vi "One_Ball_Auto.vi"(0 "Cam_Angle_To_Target":dbl=2.0715725691444784, 1 "Stopped":bool=TRUE, 2 "Dist to target":dbl=13.335309538727138, 3 "Auto_Control":T1=enum."One  Ball", 4 "Encoder_Left":dbl=-219.798918, 6 "Ultra_Sonic_Dist":dbl=31.344557836190454, 10 "Auto_Enable":bool, 14 "Yaw":dbl=63.921912939715384, 15 "Aimed?":bool) -> (18 "Intake Arm Lowered":bool, 19 "Drive_FWD Speed":dbl, 20 "Angle_Setpoint":dbl, 21 "Stage":bool, 22 "Drive_Enable":bool, 23 "Shoot":bool, 24 "Auto_Aim":bool, 25 "Rest_Encoder":bool, 26 "Rest_Gyro":bool, 27 "One_Ball_Auto":bool)   [LabVIEW 2015]
uses:
  One_Ball_Type_Def.ctl
  Auto_Selection.ctl
panel:
  in  "Ramp_Rate":dbl=1.2 format="%#_13g"
  in  "DriveForward_TIme out":i32=10000
  in  "Turning_Timeout":i32=2000
  in  "DRive to shoot time out":i32=5000
  in  "Drive_to_shoot":dbl=-0.2 format="%#_13g"
  in  "DRive_Forward_1":dbl=-1.0 format="%#_13g"
  in  "Yaw Delta Error":dbl=5.0
  in  "Max_Dist_to_Def":dbl=65.0
  in  "Min_Dist_to_Def":dbl=25.0
  out "State":T2=enum."off"
  out "error":errorcluster={"status"=TRUE, "code"=0, "source"="Drive to Shoot: Test Stop"}
  in  "Stop_DB":dbl=4.0 format="%#_13g"
  in  "Test_Stop_State":T2=enum."Drive to Shoot"
  in  "Dist_Stop_Before_Target":dbl=50.0 format="%#_13g"
  in  "Angle Turn_to_targe_DB":dbl=20.0 format="%#_13g"
  in  "Angle Turn_to_target_delta":dbl=0.5
  in  "Angle Turn_to_target":dbl=-60.0 format="%#_13g"
  in  "Dist_Low_Bar_to_Turn":dbl=160.0 format="%#_13g"
  in  "Dist_to_Lower_Arm":dbl=36.0 format="%#_13g"
  in  "Clear Error":bool
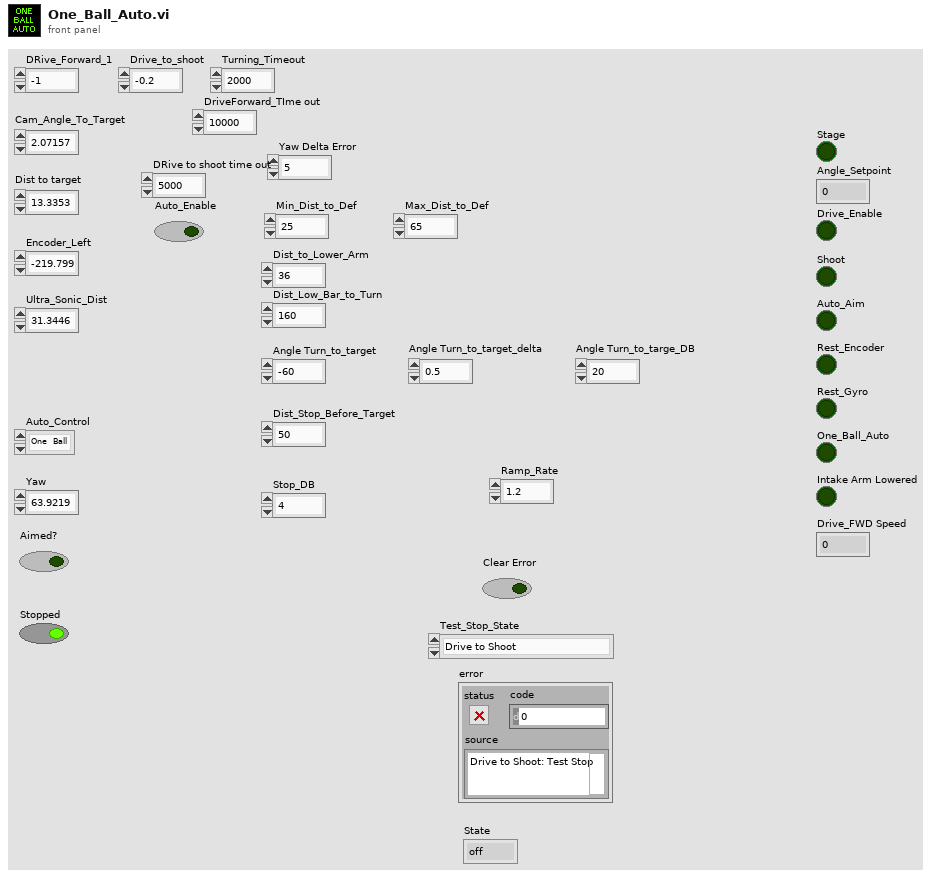
[diagram p1: front panel]
types:
  T1 = typedef "Auto_Selection.ctl" = enum16{"Low Bar", "Rough Terrain", "Rock Wall", "Ramparts", "Moat", "Cheval de Frise", "Portcullis", "None", "One  Ball", "Shoot"}
  T2 = typedef "One_Ball_Type_Def.ctl" = enum16{"Stop", "DriveForward", "LowerArm", "BeforeTeeter", "ResetOff", "ResetVar", "off", "Stop One", "Stop Two", "Tunr 60 deg", "Find Target", "Drive to Shoot", "Turn to target", "Shoot", "Stop Three", "Stop_After_Aim"}
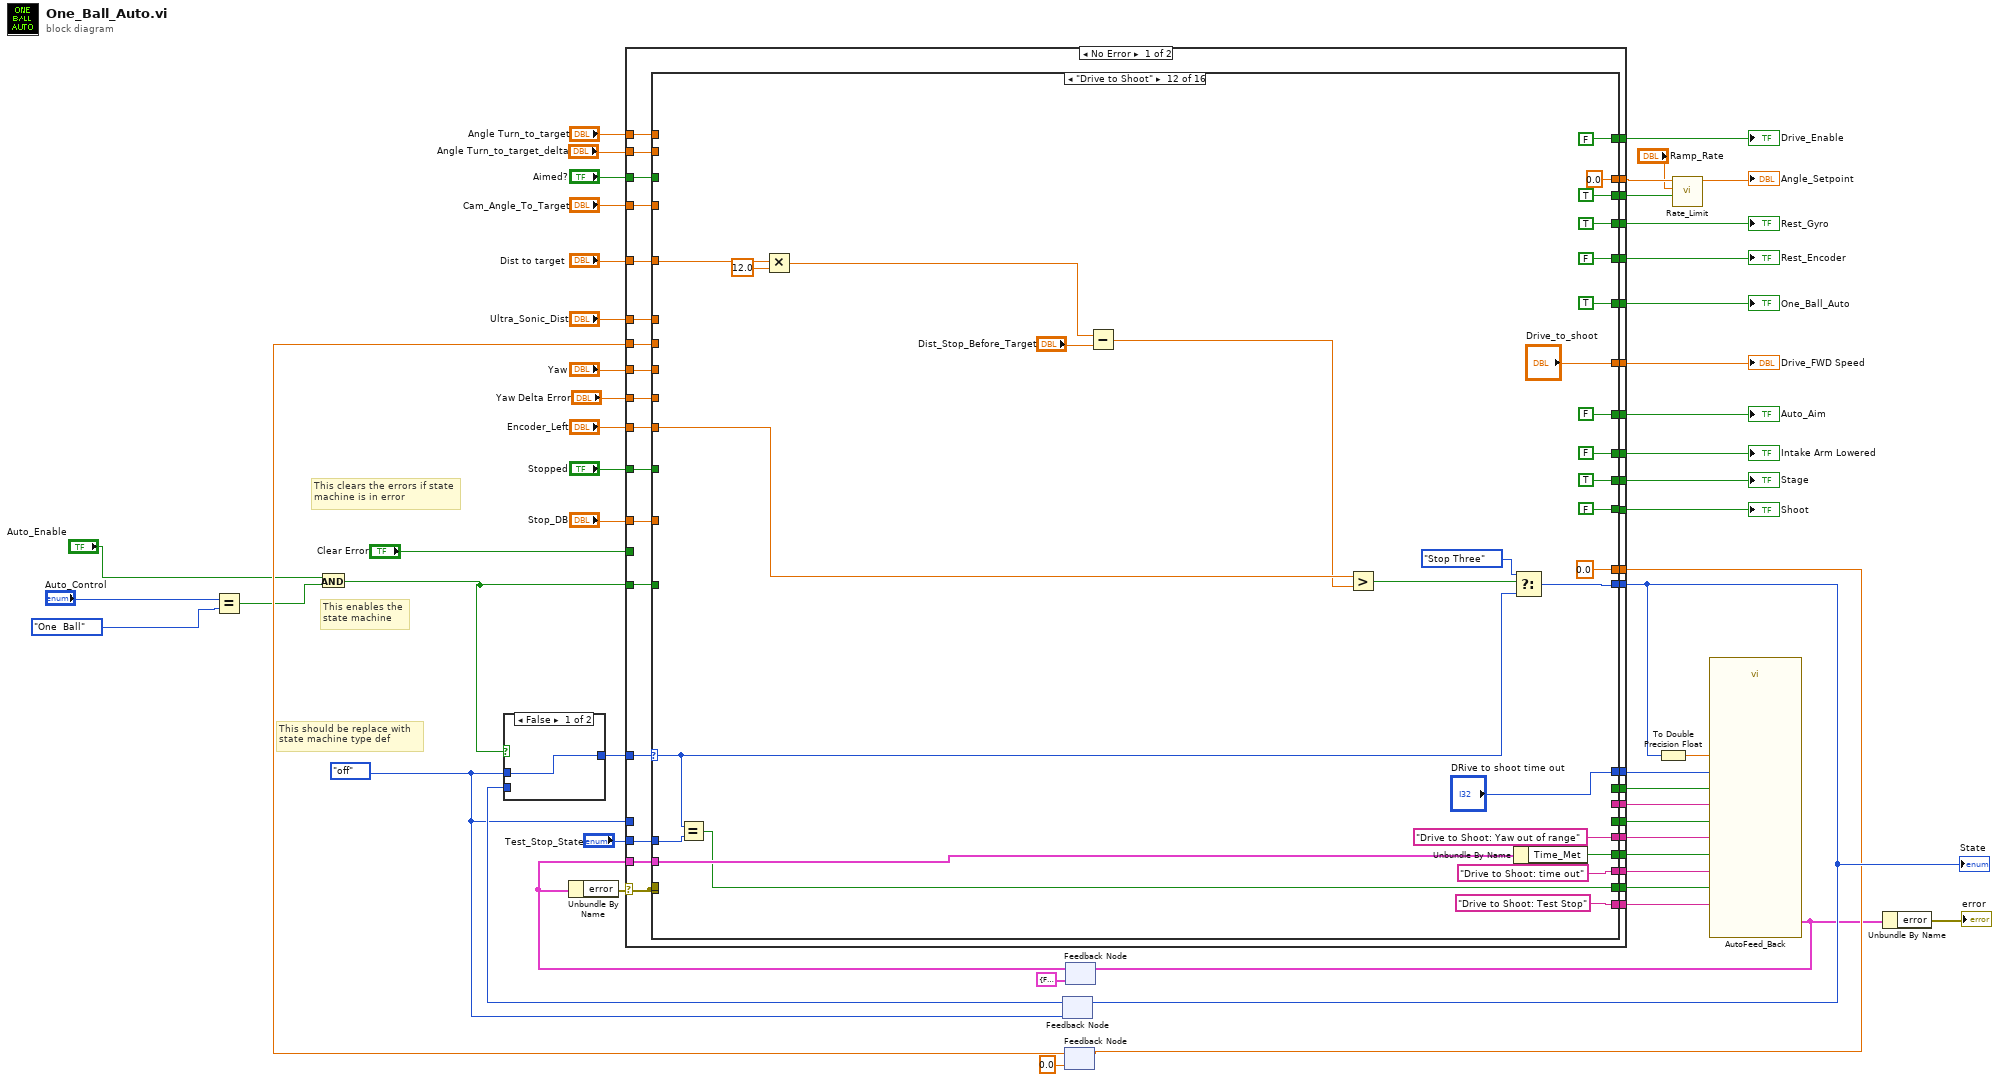
[diagram p0: block diagram]
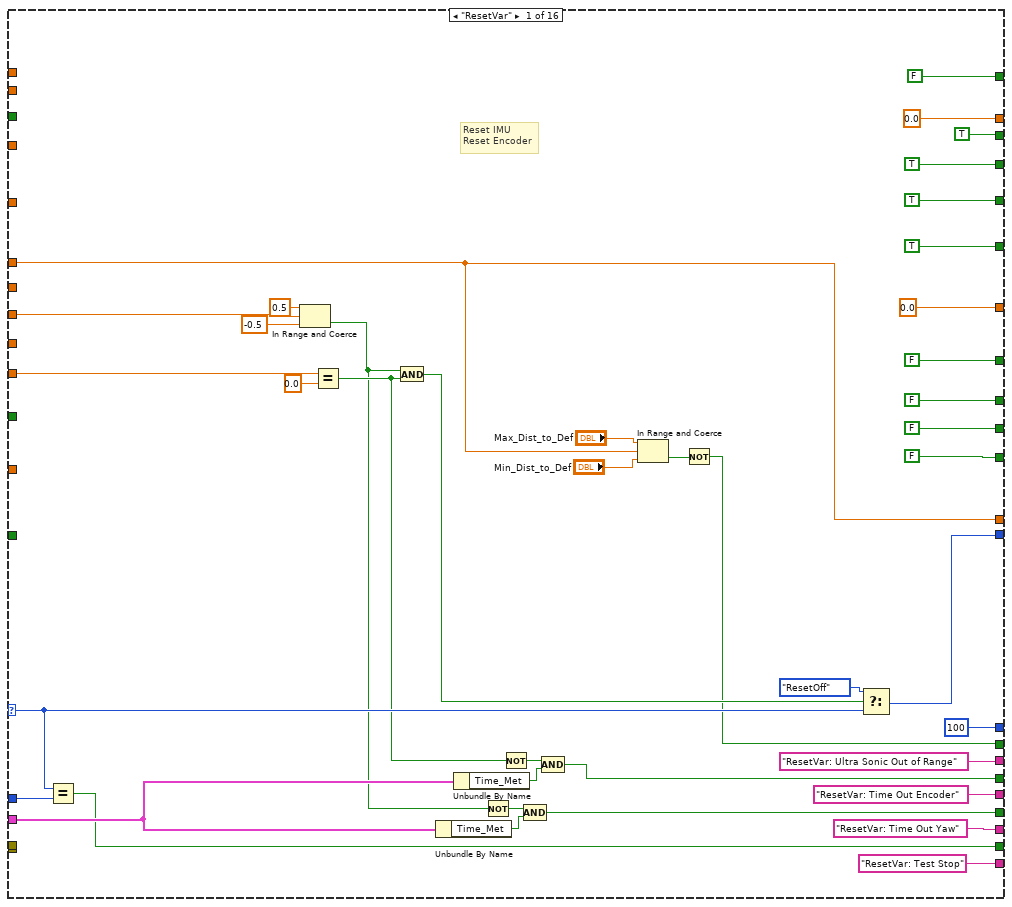
[diagram p3: hidden frame]
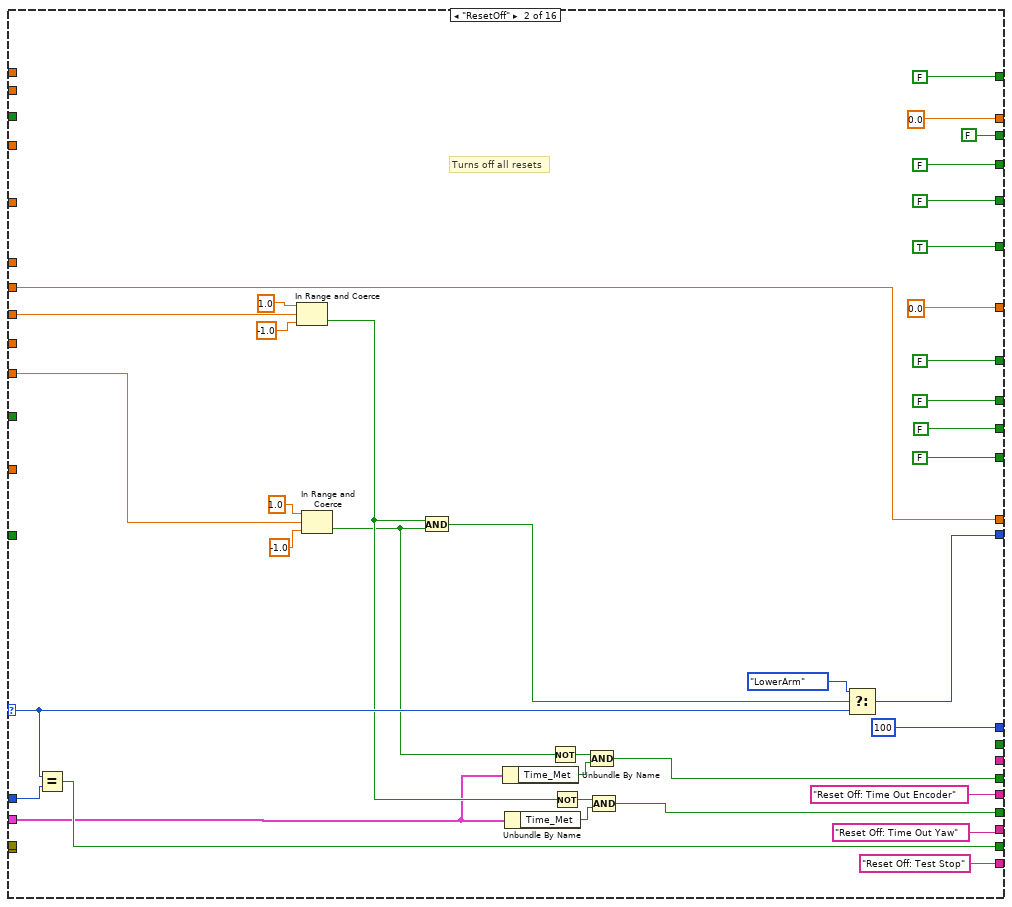
[diagram p4: hidden frame]
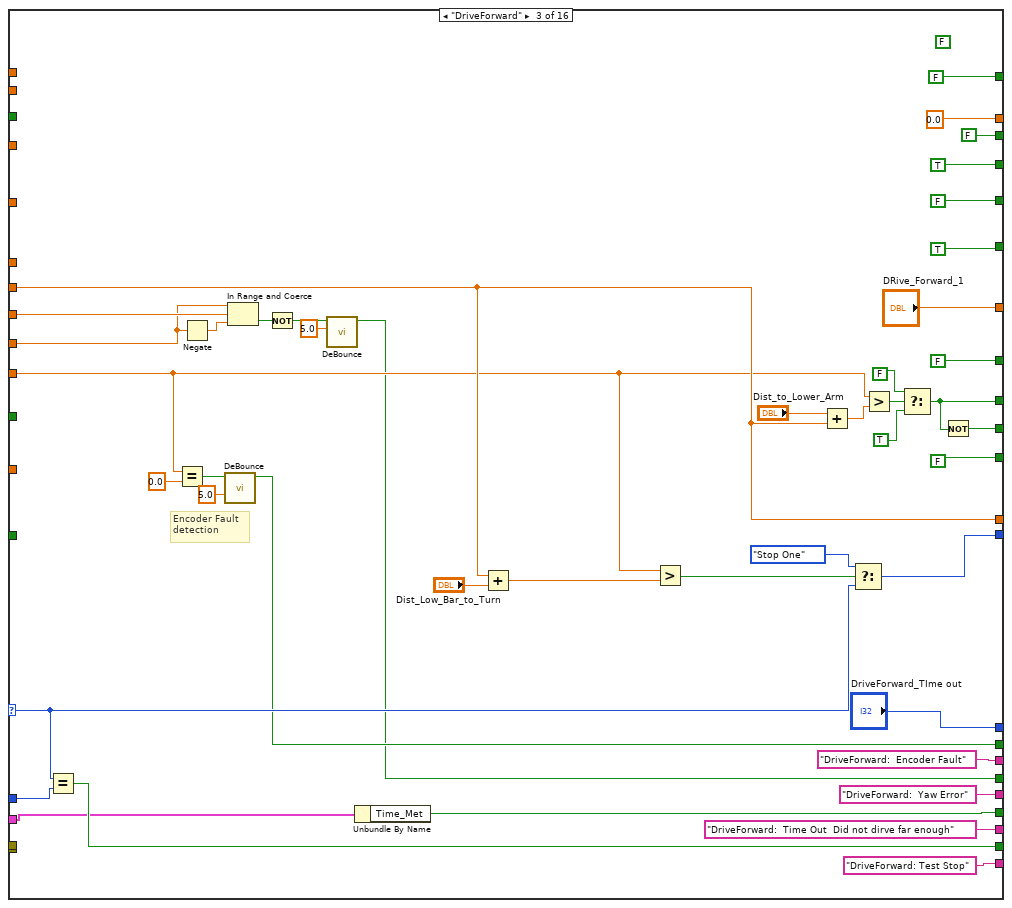
[diagram p5: hidden frame]
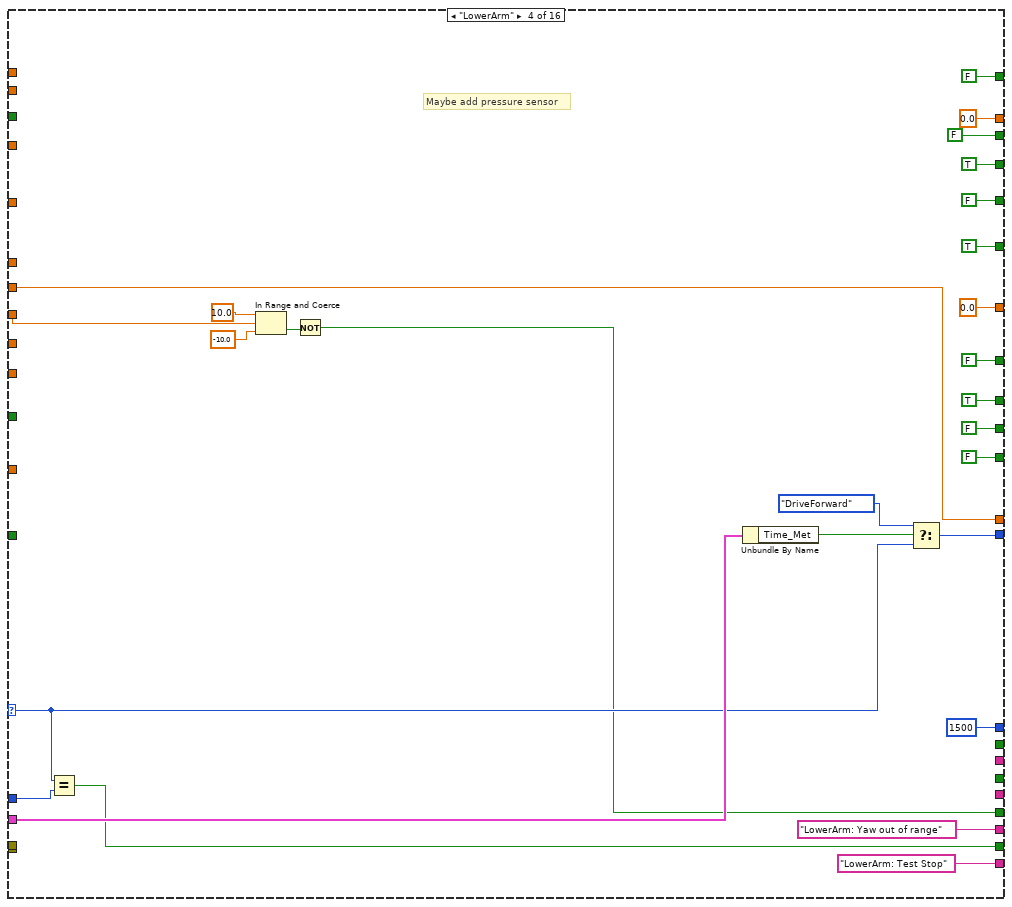
[diagram p6: hidden frame]
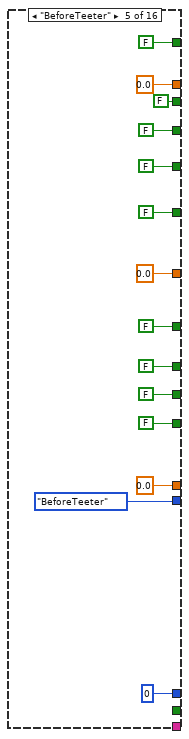
[diagram p7: hidden frame]
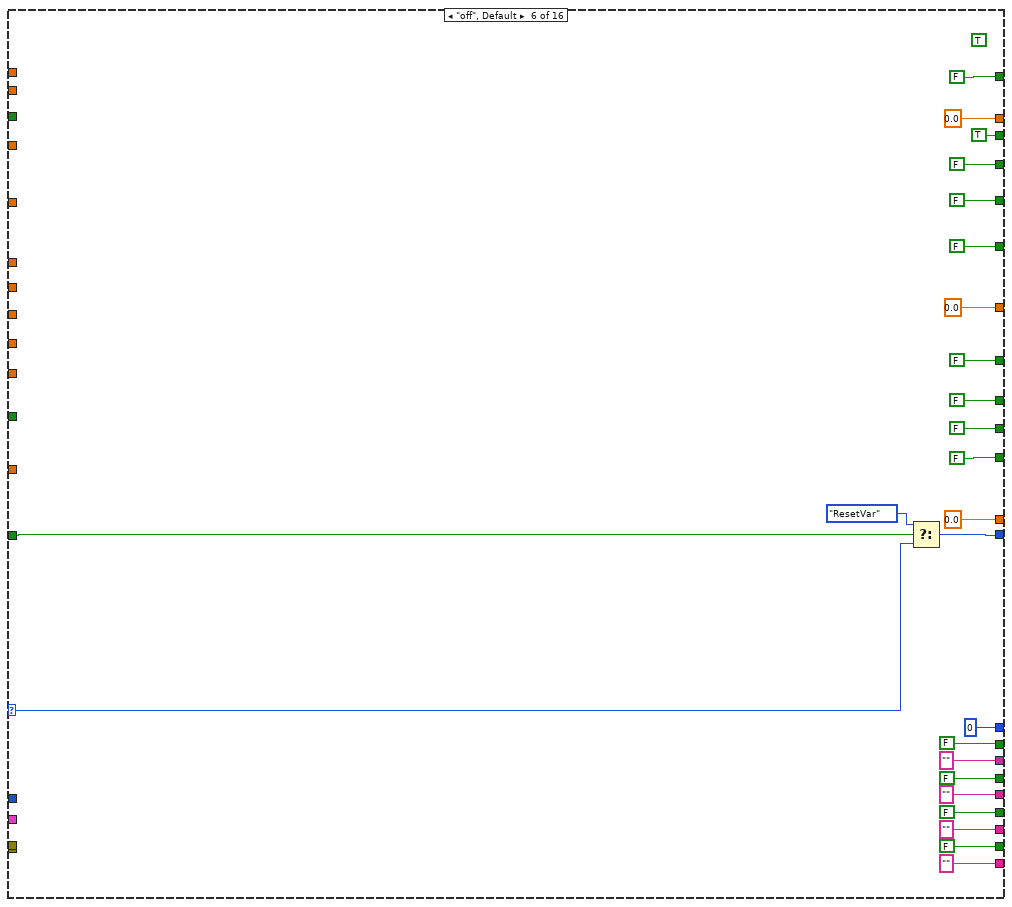
[diagram p8: hidden frame]
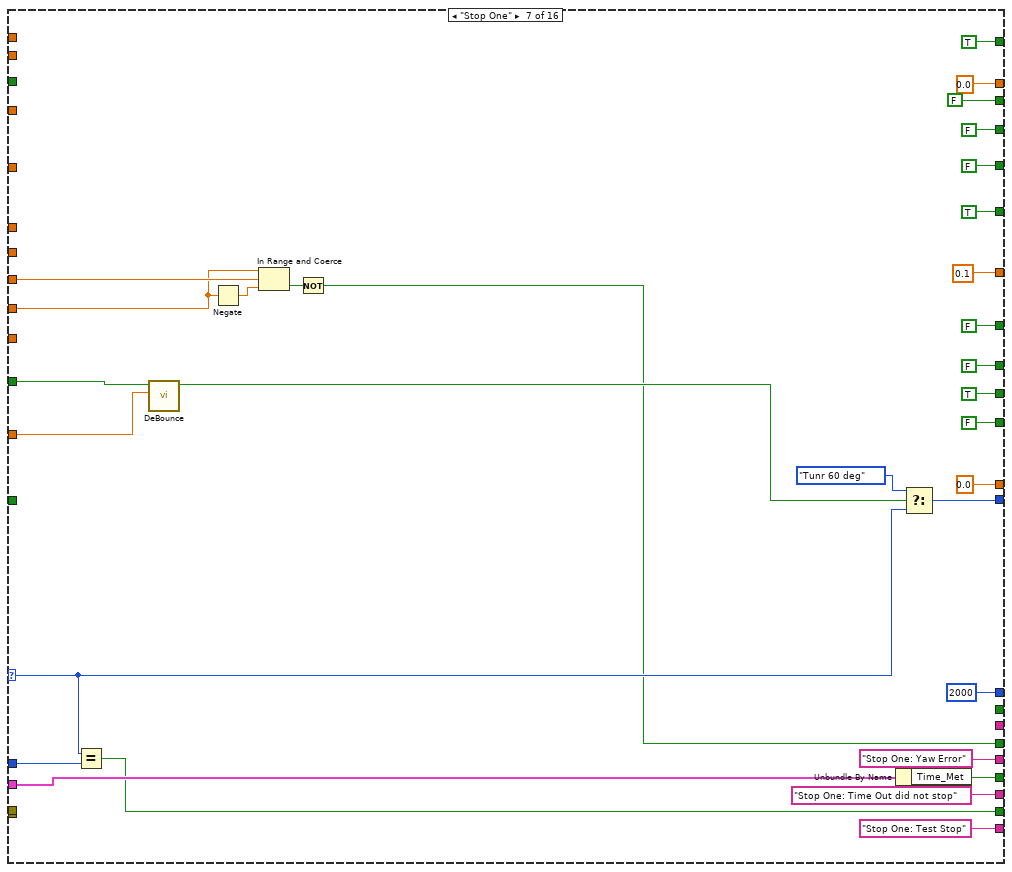
[diagram p9: hidden frame]
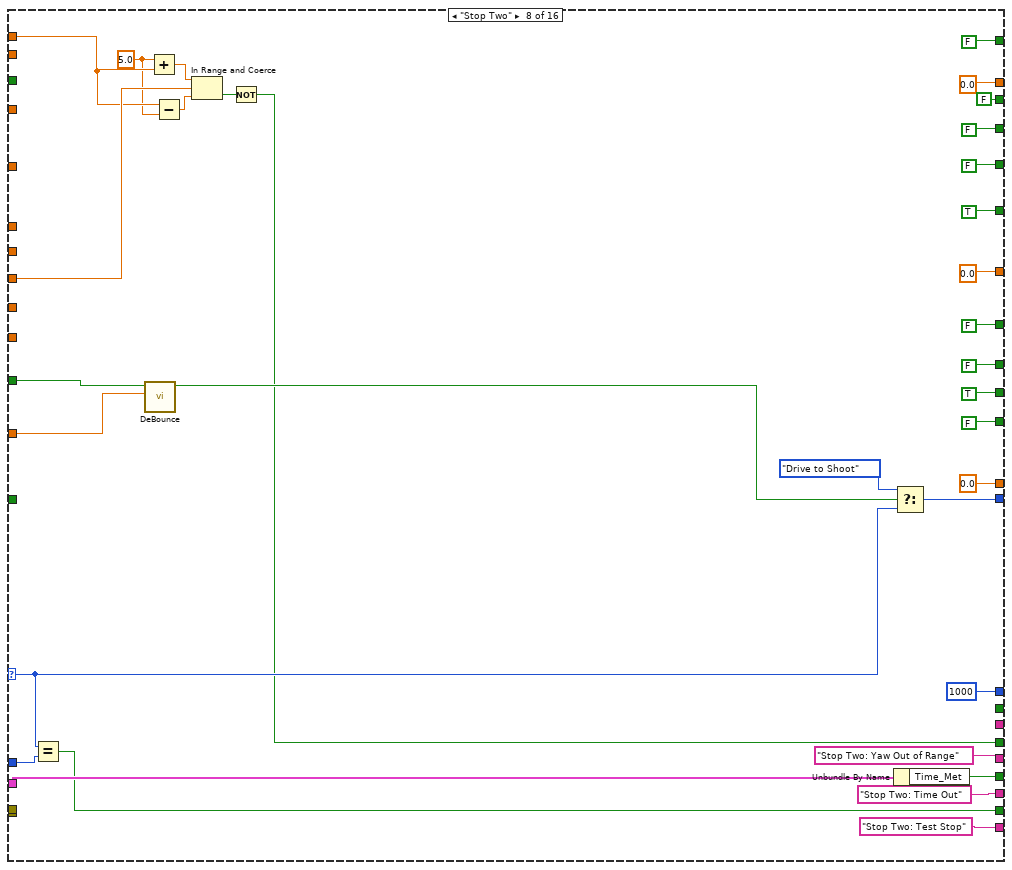
[diagram p10: hidden frame]
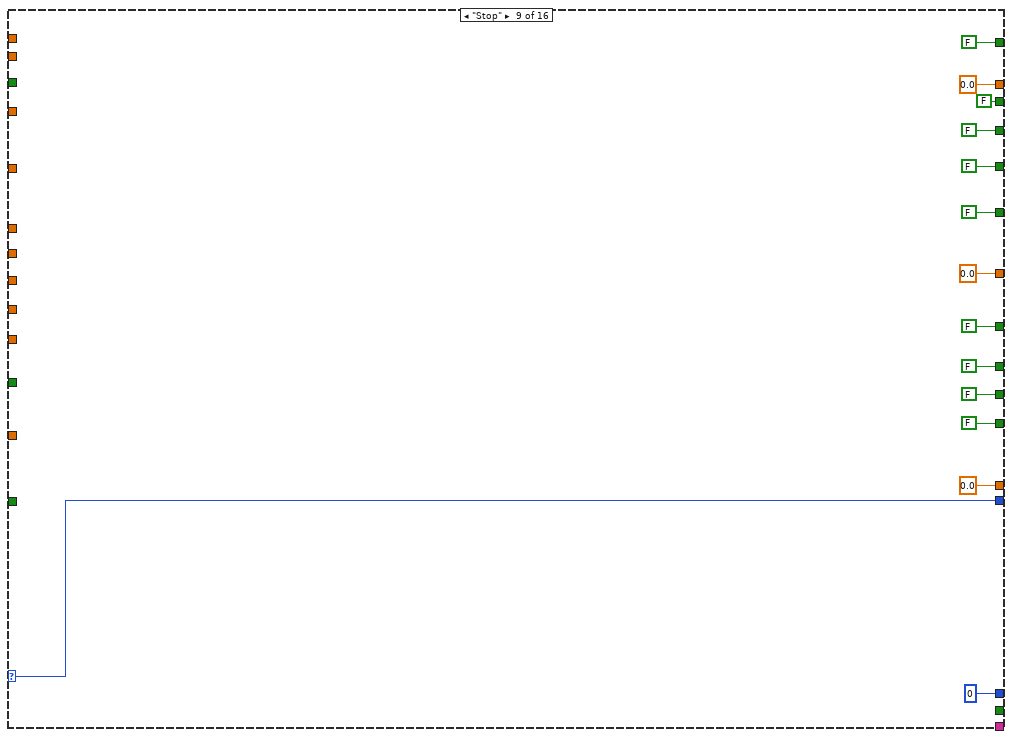
[diagram p11: hidden frame]
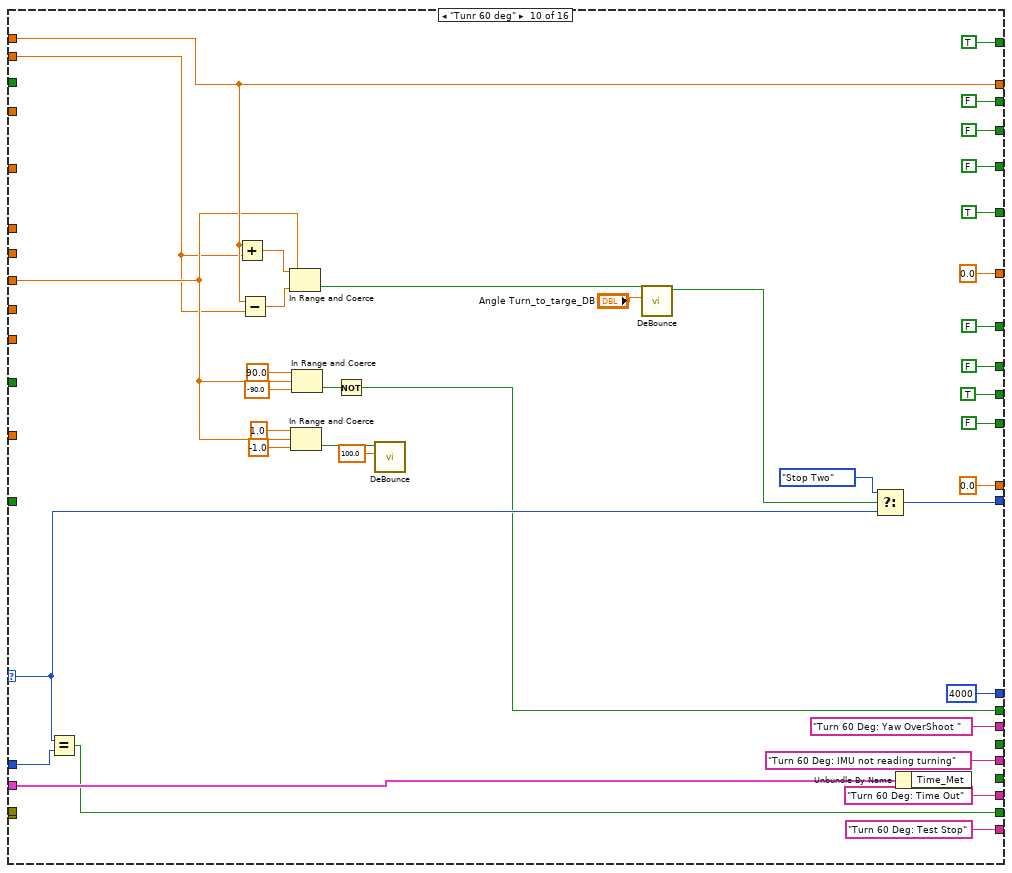
[diagram p12: hidden frame]
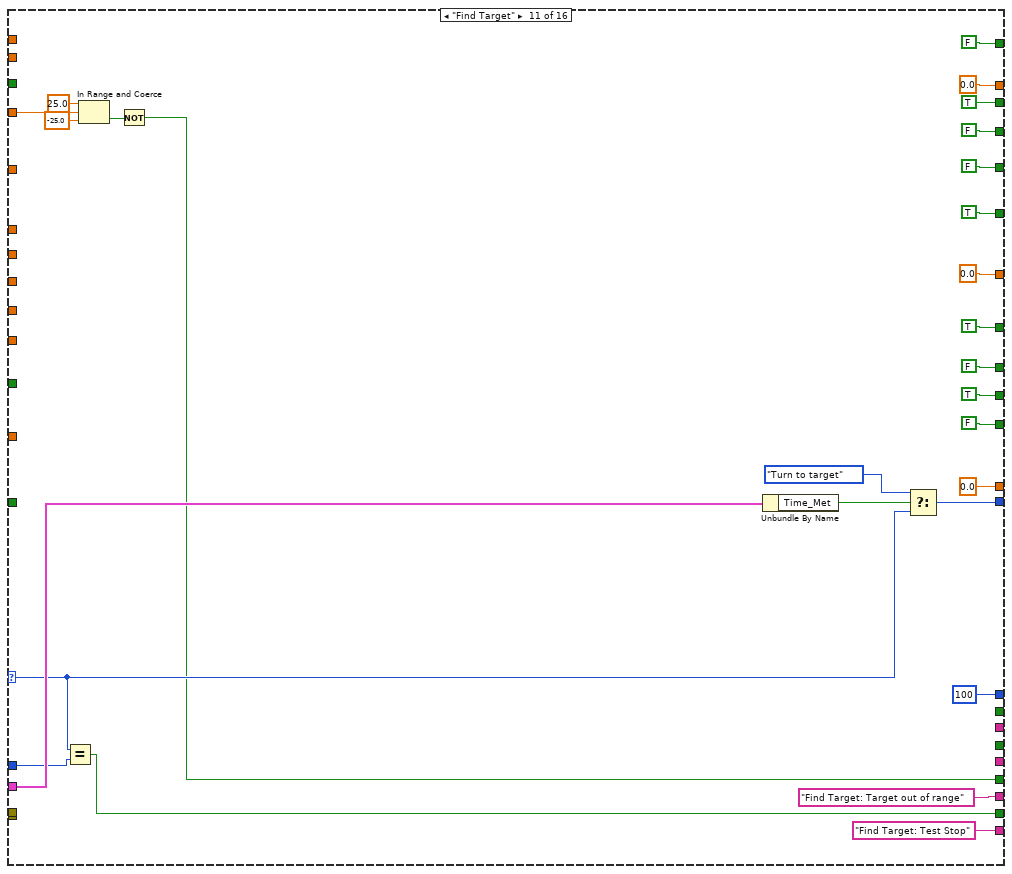
[diagram p13: hidden frame]
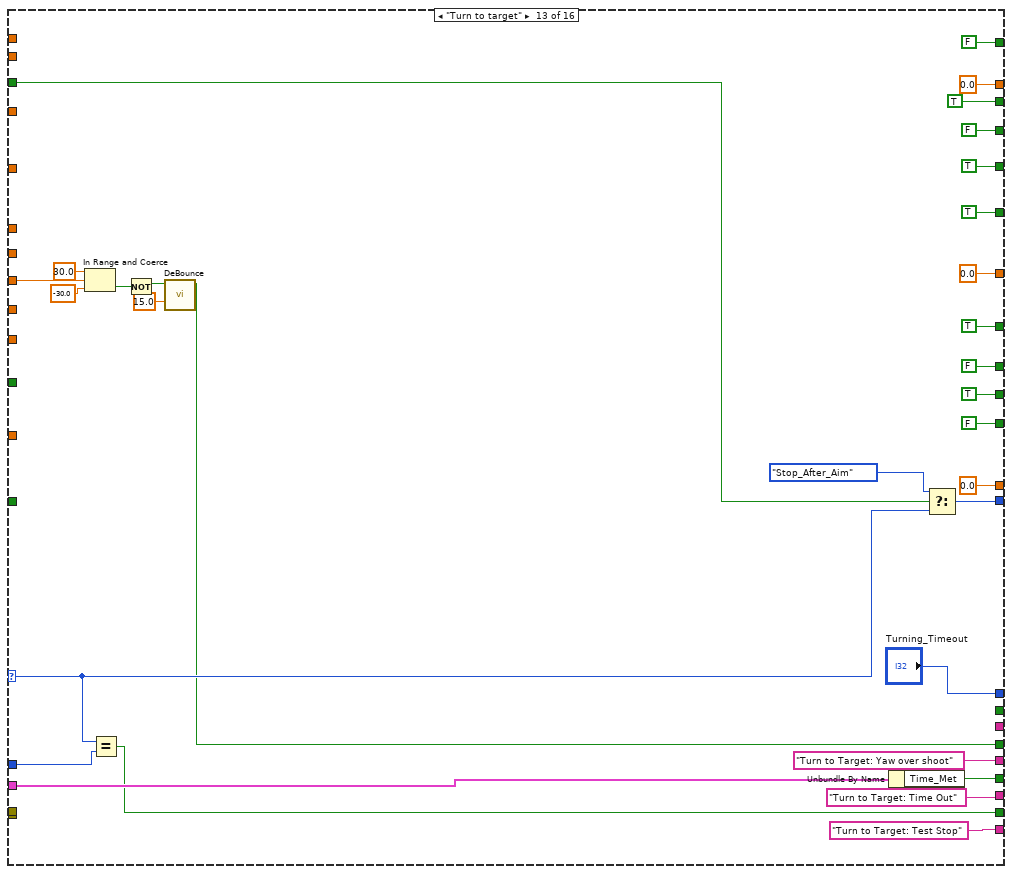
[diagram p14: hidden frame]
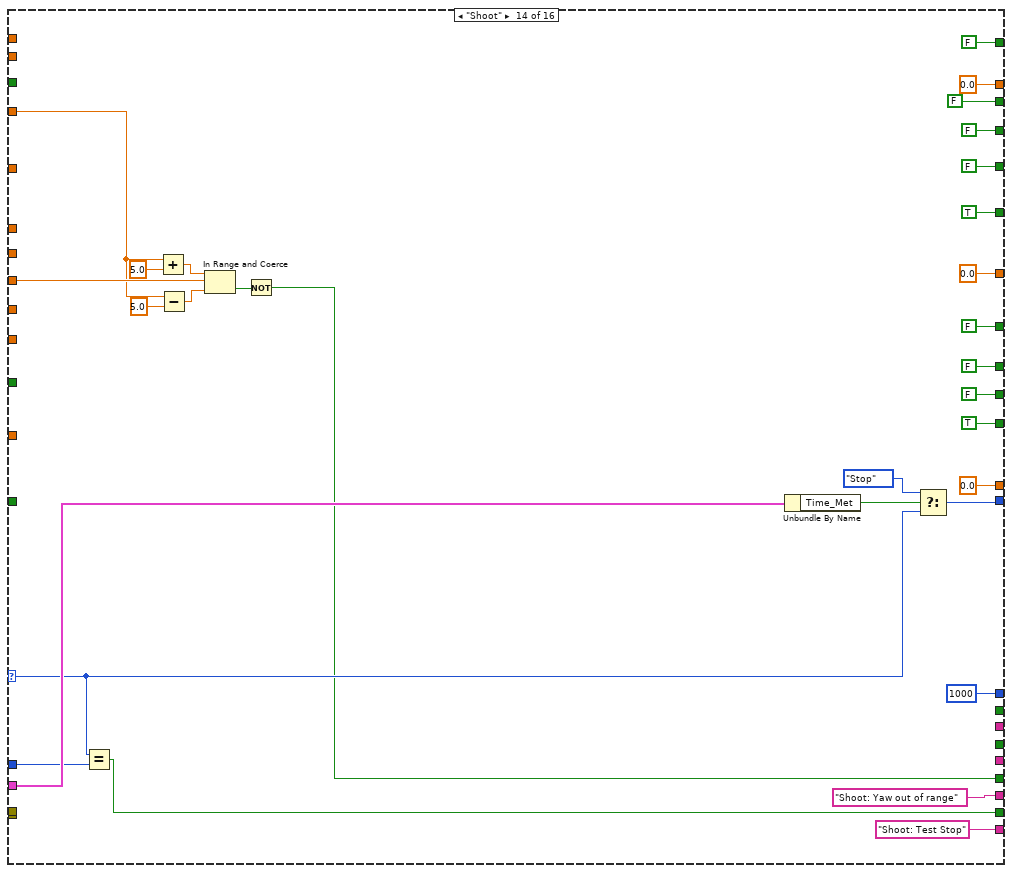
[diagram p15: hidden frame]
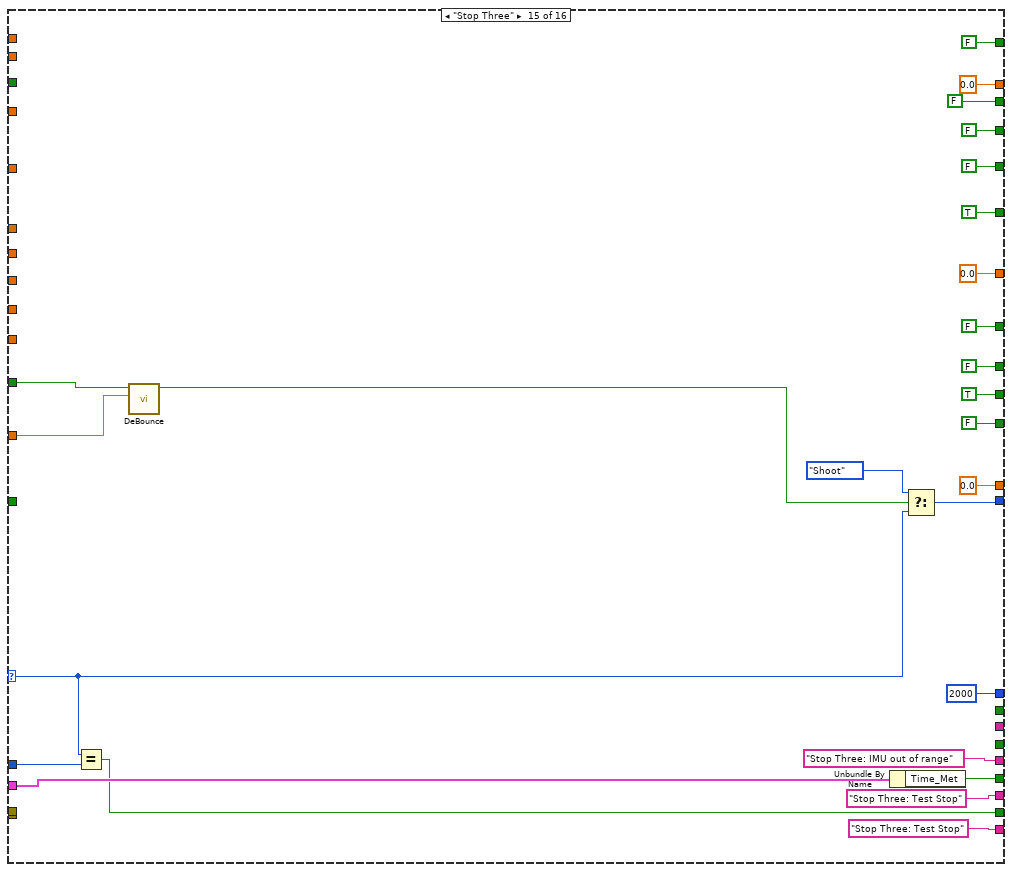
[diagram p16: hidden frame]
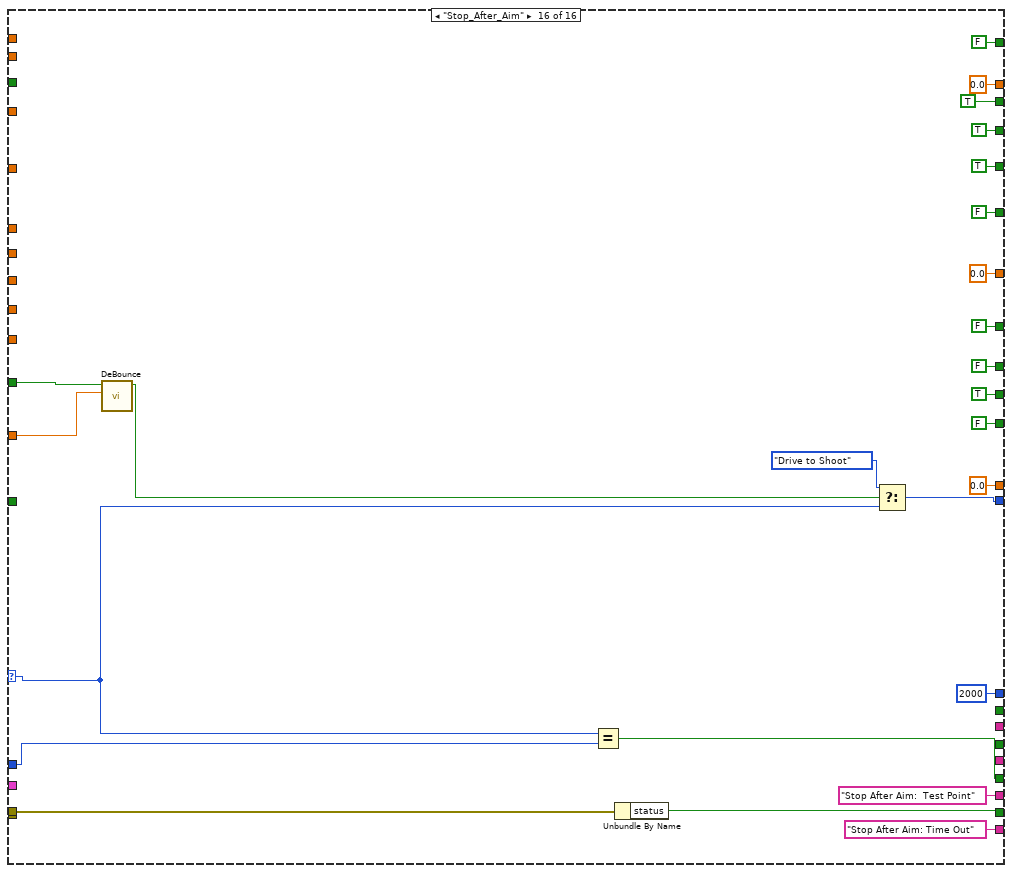
[diagram p17: hidden frame]
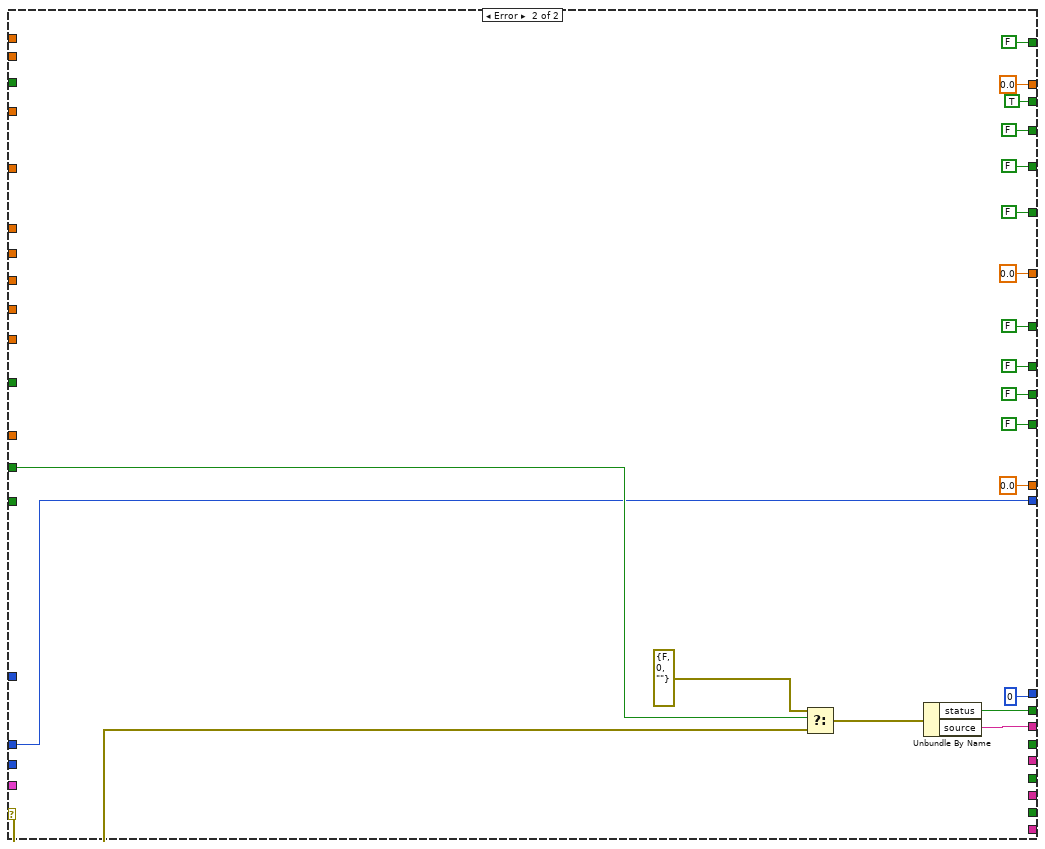
[diagram p18: hidden frame]
diagram:
  w33 = One_Ball_Type_Def."off"
  # "This clears the errors if state \nmachine is in error"
  # "This enables the \nstate machine"
  # "This should be replace with \nstate machine type def"
  n1 = Equal?(x="Auto_Control", y=Auto_Selection."One  Ball" ("Auto_Contorl.Auto_Selection 2")) -> (x = y?=w5:bool)
  n2 = And(x="Auto_Enable", y=w5) -> (x .and. y?=w3:bool)
  n3 = feedback #1(w33) -> (w45:T2)
  n4 = case shown="False" w3 {
    tunnel: w33 -> [w54 _]
    tunnel: [w54 w55] -> w46
    tunnel: w45 -> [_ w55]
    frame False {
    }
    frame True {
    }
  }
  n5 = feedback #2(0.0 ("Forward_Dist")) -> (w26:dbl)
  n6 = feedback #3(cluster{"Time_Met":bool, "error ":errorcluster} {"Time_Met"=FALSE, "error "={"status"=FALSE, "code"=0, "source"=""}} ("Feedback_State")) -> (w47:cluster{"Time_Met":bool, "error ":errorcluster})
  n7 = Unbundle By Name(w47) -> ("error"=w49:errorcluster)
  n8 = case shown="No Error" w49 {
    selector: w49 -> [w56 w572]
    tunnel: [w94 FALSE] -> w53
    tunnel: [w93 FALSE] -> w52
    tunnel: [w92 w585] -> w38
    tunnel: [w91 0] -> w51
    tunnel: "Clear Error" -> [_ w586]
    tunnel: w47 -> [w90 _]
    tunnel: w3 -> [w89 _]
    tunnel: w46 -> [w78 _]
    tunnel: w33 -> [_ w585]
    tunnel: [w88 0.0] -> w43
    tunnel: [w87 FALSE] -> w42
    tunnel: [w86 FALSE] -> w41
    tunnel: "Yaw" -> [w85 _]
    tunnel: "Encoder_Left" -> [w84 _]
    tunnel: [w83 FALSE] -> w37
    tunnel: [w82 FALSE] -> w36
    tunnel: "Ultra_Sonic_Dist" -> [w81 _]
    tunnel: [w80 0.0 ("Forward_Dist")] -> w22
    tunnel: w26 -> [w79 _]
    tunnel: [w77 0.0 ("Angle Turn_to_target")] -> w2
    tunnel: [w76 FALSE] -> w32
    tunnel: [w75 FALSE] -> w31
    tunnel: "Dist to target" -> [w74 _]
    tunnel: "Cam_Angle_To_Target" -> [w73 _]
    tunnel: "Aimed?" -> [w72 _]
    tunnel: "Angle Turn_to_target" -> [w71 _]
    tunnel: "Test_Stop_State" -> [w70 _]
    tunnel: "Stopped" -> [w69 _]
    tunnel: "Stop_DB" -> [w68 _]
    tunnel: [w67 w570] -> w21
    tunnel: [w66 _] -> w20
    tunnel: [w65 _] -> w19
    tunnel: [w64 _] -> w18
    tunnel: [w63 w569] -> w17
    tunnel: [w62 _] -> w16
    tunnel: [w61 _] -> w15
    tunnel: [w60 _] -> w14
    tunnel: "Yaw Delta Error" -> [w59 _]
    tunnel: "Angle Turn_to_target_delta" -> [w58 _]
    tunnel: [w57 TRUE] -> w6
    frame No Error {
      n9 = case shown="\"Drive to Shoot\"" w78 {
        selector: w78 -> [w119 w150 w194 w227 _ w267 w298 w331 w348 w378 w408 w436 w470 w500 w527 w545]
        tunnel: [TRUE FALSE TRUE TRUE FALSE FALSE FALSE FALSE FALSE FALSE FALSE TRUE FALSE FALSE FALSE TRUE] -> w94
        tunnel: [TRUE FALSE FALSE FALSE FALSE FALSE FALSE FALSE FALSE FALSE FALSE FALSE TRUE FALSE FALSE TRUE] -> w93
        tunnel: [100 100 "DriveForward_TIme out" 1500 0 0 2000 1000 0 4000 100 "DRive to shoot time out" "Turning_Timeout" 1000 2000 2000 ("Turning_Timeout")] -> w91
        tunnel: [w130 w167 w211 w236 One_Ball_Type_Def."BeforeTeeter" w277 w305 w335 w348 w389 w414 w445 w475 w504 w531 w552] -> w92
        tunnel: w90 -> [w113 w140 w188 w233 _ _ w302 w330 _ w385 w411 w438 w472 w502 w526 _]
        tunnel: w56 -> [_ _ _ _ _ _ _ _ _ _ _ _ _ _ _ _]
        tunnel: w89 -> [_ _ _ _ _ w275 _ _ _ _ _ _ _ _ _ _]
        tunnel: [0.0 0.0 "DRive_Forward_1" 0.0 0.0 0.0 0.1 0.0 0.0 0.0 0.0 "Drive_to_shoot" 0.0 0.0 0.0 0.0 ("Drive_to_shoot")] -> w88
        tunnel: [TRUE TRUE TRUE TRUE FALSE FALSE TRUE TRUE FALSE TRUE TRUE TRUE TRUE TRUE TRUE FALSE] -> w87
        tunnel: [FALSE FALSE w195 TRUE FALSE FALSE FALSE FALSE FALSE FALSE FALSE FALSE FALSE FALSE FALSE FALSE] -> w86
        tunnel: w85 -> [w98 w162 w187 w222 _ _ w288 w323 _ w368 _ _ w465 w491 _ _]
        tunnel: w84 -> [w128 w161 w182 _ _ _ _ _ _ _ _ w442 _ _ _ _]
        tunnel: [FALSE FALSE FALSE FALSE FALSE FALSE FALSE FALSE FALSE FALSE FALSE FALSE FALSE TRUE FALSE FALSE] -> w83
        tunnel: [FALSE FALSE FALSE FALSE FALSE FALSE FALSE FALSE FALSE FALSE TRUE FALSE TRUE FALSE FALSE FALSE] -> w82
        tunnel: w81 -> [w106 _ _ _ _ _ _ _ _ _ _ _ _ _ _ _]
        tunnel: [w106 w156 w200 w231 0.0 ("Forward_Dist") 0.0 ("Forward_Dist") 0.0 ("Forward_Dist") 0.0 ("Forward_Dist") 0.0 ("Forward_Dist") 0.0 ("Forward_Dist") 0.0 ("Forward_Dist") 0.0 ("Forward_Dist") 0.0 ("Forward_Dist") 0.0 ("Forward_Dist") 0.0 ("Forward_Dist") 0.0 ("Forward_Dist")] -> w80
        tunnel: w79 -> [_ w156 w200 w231 _ _ _ _ _ _ _ _ _ _ _ _]
        tunnel: [0.0 0.0 0.0 0.0 0.0 ("Angle Turn_to_target") 0.0 0.0 0.0 ("Angle Turn_to_target") 0.0 ("Angle Turn_to_target") w379 0.0 ("Angle Turn_to_target") 0.0 ("Angle Turn_to_target") 0.0 ("Angle Turn_to_target") 0.0 ("Angle Turn_to_target") 0.0 ("Angle Turn_to_target") 0.0 ("Angle Turn_to_target")] -> w77
        tunnel: [FALSE FALSE FALSE FALSE FALSE FALSE TRUE FALSE FALSE TRUE FALSE FALSE FALSE FALSE FALSE FALSE] -> w76
        tunnel: [FALSE FALSE w196 FALSE FALSE FALSE TRUE TRUE FALSE TRUE TRUE TRUE TRUE FALSE TRUE TRUE] -> w75
        tunnel: w74 -> [_ _ _ _ _ _ _ _ _ _ _ w429 _ _ _ _]
        tunnel: w73 -> [_ _ _ _ _ _ _ _ _ _ w405 _ _ w490 _ _]
        tunnel: w72 -> [_ _ _ _ _ _ _ _ _ _ _ _ w471 _ _ _]
        tunnel: w71 -> [_ _ _ _ _ _ _ w320 _ w379 _ _ _ _ _ _]
        tunnel: w70 -> [w118 w151 w193 w226 _ _ w297 w332 _ w377 w409 w437 w469 w499 w528 w546]
        tunnel: w69 -> [_ _ _ _ _ _ w284 w315 _ _ _ _ _ _ w518 w555]
        tunnel: w68 -> [_ _ _ _ _ _ w295 w329 _ _ _ _ _ _ w525 w554]
        tunnel: [w104 _ w178 _ _ FALSE _ _ _ w365 _ _ _ _ _ _] -> w67
        tunnel: [w110 w138 w175 _ _ FALSE w287 w317 _ _ _ _ w458 _ _ _] -> w66
        tunnel: [w111 w144 w192 w218 _ FALSE w292 w324 _ _ w401 w433 w456 w489 w520 w544] -> w65
        tunnel: [w102 w149 w189 w225 _ FALSE w294 w327 _ w376 w407 w435 w468 w498 w523 w548] -> w64
        tunnel: ["ResetVar: Ultra Sonic Out of Range" ("source") _ "DriveForward:  Encoder Fault" ("source") _ _ "" _ _ _ "Turn 60 Deg: Yaw OverShoot " ("source") _ _ _ _ _ _] -> w63
        tunnel: ["ResetVar: Time Out Encoder" ("source") "Reset Off: Time Out Encoder" ("source") "DriveForward:  Yaw Error" ("source") _ _ "" "Stop One: Yaw Error" ("source") "Stop Two: Yaw Out of Range" ("source") _ "Turn 60 Deg: IMU not reading turning" ("source") _ "Drive to Shoot: Yaw out of range" ("source") "Turn to Target: Yaw over shoot" ("source") _ "Stop Three: IMU out of range" ("source") _] -> w62
        tunnel: ["ResetVar: Time Out Yaw" ("source") "Reset Off: Time Out Yaw" ("source") "DriveForward:  Time Out  Did not dirve far enough" ("source") "LowerArm: Yaw out of range" ("source") _ "" "Stop One: Time Out did not stop" ("source") "Stop Two: Time Out" ("source") _ "Turn 60 Deg: Time Out" ("source") "Find Target: Target out of range" ("source") "Drive to Shoot: time out" ("source") "Turn to Target: Time Out" ("source") "Shoot: Yaw out of range" ("source") "Stop Three: Test Stop" ("source") "Stop After Aim:  Test Point" ("source")] -> w61
        tunnel: ["ResetVar: Test Stop" ("source") "Reset Off: Test Stop" ("source") "DriveForward: Test Stop" ("source") "LowerArm: Test Stop" ("source") _ "" "Stop One: Test Stop" ("source") "Stop Two: Test Stop" ("source") _ "Turn 60 Deg: Test Stop" ("source") "Find Target: Test Stop" ("source") "Drive to Shoot: Test Stop" ("source") "Turn to Target: Test Stop" ("source") "Shoot: Test Stop" ("source") "Stop Three: Test Stop" ("source") "Stop After Aim: Time Out" ("source")] -> w60
        tunnel: w59 -> [_ _ w183 _ _ _ w285 _ _ _ _ _ _ _ _ _]
        tunnel: w58 -> [_ _ _ _ _ _ _ _ _ w362 _ _ _ _ _ _]
        tunnel: [TRUE FALSE FALSE FALSE FALSE TRUE FALSE FALSE FALSE FALSE TRUE TRUE TRUE FALSE FALSE TRUE] -> w57
        tunnel: w56 -> [_ _ _ _ _ _ _ _ _ _ _ _ _ _ _ w549]
        frame "ResetVar" {
          # "Reset IMU\nReset Encoder"
          n10 = Equal?(x=w119, y=w118) -> (x = y?=w102:bool)
          n11 = In Range and Coerce(upper limit=0.5, x=w98, lower limit=-0.5) -> (In Range?=w99:bool)  [unwired: 1 out]
          n12 = Equal?(x=w128, y=0.0) -> (x = y?=w112:bool)
          n13 = And(x=w99, y=w112) -> (x .and. y?=w127:bool)
          n14 = Unbundle By Name(w113) -> ("Time_Met"=w116:bool)
          n15 = Unbundle By Name(w113) -> ("Time_Met"=w115:bool)
          n16 = Not(x=w99) -> (.not. x?=w117:bool)
          n17 = Not(x=w112) -> (.not. x?=w114:bool)
          n18 = Compound Arithmetic op=AND(w117, w116) -> (w111:bool)
          n19 = Compound Arithmetic op=AND(w114, w115) -> (w110:bool)
          n20 = In Range and Coerce(upper limit="Max_Dist_to_Def", x=w106, lower limit="Min_Dist_to_Def") -> (In Range?=w105:bool)  [unwired: 1 out]
          n21 = Not(x=w105) -> (.not. x?=w104:bool)
          n22 = Select(t=One_Ball_Type_Def."ResetOff", s=w127, f=w119) -> (s? t:f=w130:T2)
        }
        frame "ResetOff" {
          # "Turns off all resets"
          n23 = Equal?(x=w150, y=w151) -> (x = y?=w149:bool)
          n24 = In Range and Coerce(upper limit=1.0, x=w162, lower limit=-1.0) -> (In Range?=w143:bool)  [unwired: 1 out]
          n25 = In Range and Coerce(upper limit=1.0, x=w161, lower limit=-1.0) -> (In Range?=w139:bool)  [unwired: 1 out]
          n26 = And(x=w143, y=w139) -> (x .and. y?=w160:bool)
          n27 = Unbundle By Name(w140) -> ("Time_Met"=w142:bool)
          n28 = Unbundle By Name(w140) -> ("Time_Met"=w147:bool)
          n29 = Not(x=w139) -> (.not. x?=w141:bool)
          n30 = Not(x=w143) -> (.not. x?=w146:bool)
          n31 = Compound Arithmetic op=AND(w141, w142) -> (w138:bool)
          n32 = Compound Arithmetic op=AND(w146, w147) -> (w144:bool)
          n33 = Select(t=One_Ball_Type_Def."LowerArm", s=w160, f=w150) -> (s? t:f=w167:T2)
        }
        frame "DriveForward" {
          (unwired) FALSE
          # "Encoder Fault \ndetection"
          n34 = Equal?(x=w194, y=w193) -> (x = y?=w189:bool)
          n35 = Equal?(x=w182, y=0.0) -> (x = y?=w180:bool)
          n36 = Negate(x=w183) -> (-x=w186:dbl)
          n37 = call "DeBounce.vi"("DB_Count"=5.0, "Value"=w180) -> ("BD_Value"=w178:bool)  [unwired: 9 in]
          n38 = In Range and Coerce(upper limit=w183, x=w187, lower limit=w186) -> (In Range?=w185:bool)  [unwired: 1 out]
          n39 = Not(x=w185) -> (.not. x?=w174:bool)
          n40 = call "DeBounce.vi"("DB_Count"=5.0, "Value"=w174) -> ("BD_Value"=w175:bool)  [unwired: 9 in]
          n41 = Unbundle By Name(w188) -> ("Time_Met"=w192:bool)
          n42 = Add(x=w200, y="Dist_Low_Bar_to_Turn") -> (x+y=w199:dbl)
          n43 = Greater?(x=w182, y=w199) -> (0:w202:bool)
          n44 = Add(x="Dist_to_Lower_Arm", y=w200) -> (x+y=w206:dbl)
          n45 = Select(t=One_Ball_Type_Def."Stop One", s=w202, f=w194) -> (s? t:f=w211:T2)
          n46 = Greater?(x=w182, y=w206) -> (0:w207:bool)
          n47 = Select(t=FALSE, s=w207, f=TRUE) -> (s? t:f=w195:bool)
          n48 = Not(x=w195) -> (.not. x?=w196:bool)
        }
        frame "LowerArm" {
          # "Maybe add pressure sensor"
          n49 = Equal?(x=w227, y=w226) -> (x = y?=w225:bool)
          n50 = In Range and Coerce(upper limit=10.0, x=w222, lower limit=-10.0) -> (In Range?=w219:bool)  [unwired: 1 out]
          n51 = Not(x=w219) -> (.not. x?=w218:bool)
          n52 = Unbundle By Name(w233) -> ("Time_Met"=w232:bool)
          n53 = Select(t=One_Ball_Type_Def."DriveForward", s=w232, f=w227) -> (s? t:f=w236:T2)
        }
        frame "BeforeTeeter" {
        }
        frame "off", Default {
          (unwired) TRUE
          n54 = Select(t=One_Ball_Type_Def."ResetVar", s=w275, f=w267) -> (s? t:f=w277:T2)
        }
        frame "Stop One" {
          n55 = Equal?(x=w298, y=w297) -> (x = y?=w294:bool)
          n56 = call "DeBounce.vi"("DB_Count"=w295, "Value"=w284) -> ("BD_Value"=w296:bool)  [unwired: 9 in]
          n57 = Negate(x=w285) -> (-x=w290:dbl)
          n58 = In Range and Coerce(upper limit=w285, x=w288, lower limit=w290) -> (In Range?=w289:bool)  [unwired: 1 out]
          n59 = Not(x=w289) -> (.not. x?=w287:bool)
          n60 = Unbundle By Name(w302) -> ("Time_Met"=w292:bool)
          n61 = Select(t=One_Ball_Type_Def."Tunr 60 deg", s=w296, f=w298) -> (s? t:f=w305:T2)
        }
        frame "Stop Two" {
          w319 = 5.0 ("x")
          n62 = Equal?(x=w331, y=w332) -> (x = y?=w327:bool)
          n63 = call "DeBounce.vi"("DB_Count"=w329, "Value"=w315) -> ("BD_Value"=w328:bool)  [unwired: 9 in]
          n64 = Add(x=w319, y=w320) -> (x+y=w322:dbl)
          n65 = Subtract(x=w320, y=w319) -> (x-y=w321:dbl)
          n66 = In Range and Coerce(upper limit=w322, x=w323, lower limit=w321) -> (In Range?=w318:bool)  [unwired: 1 out]
          n67 = Not(x=w318) -> (.not. x?=w317:bool)
          n68 = Unbundle By Name(w330) -> ("Time_Met"=w324:bool)
          n69 = Select(t=One_Ball_Type_Def."Drive to Shoot", s=w328, f=w331) -> (s? t:f=w335:T2)
        }
        frame "Stop" {
        }
        frame "Tunr 60 deg" {
          n70 = Equal?(x=w378, y=w377) -> (x = y?=w376:bool)
          n71 = Add(x=w379, y=w362) -> (x+y=w384:dbl)
          n72 = Subtract(x=w379, y=w362) -> (x-y=w383:dbl)
          n73 = In Range and Coerce(upper limit=w384, x=w368, lower limit=w383) -> (In Range?=w382:bool)  [unwired: 1 out]
          n74 = In Range and Coerce(upper limit=1.0, x=w368, lower limit=-1.0) -> (In Range?=w364:bool)  [unwired: 1 out]
          n75 = In Range and Coerce(upper limit=90.0, x=w368, lower limit=-90.0) -> (In Range?=w366:bool)  [unwired: 1 out]
          n76 = Not(x=w366) -> (.not. x?=w365:bool)
          n77 = call "DeBounce.vi"("DB_Count"=100.0, "Value"=w364) -> ()  [unwired: 9 in, 1 out]
          n78 = call "DeBounce.vi"("DB_Count"="Angle Turn_to_targe_DB", "Value"=w382) -> ("BD_Value"=w380:bool)  [unwired: 9 in]
          n79 = Select(t=One_Ball_Type_Def."Stop Two", s=w380, f=w378) -> (s? t:f=w389:T2)
          n80 = Unbundle By Name(w385) -> ()  [unwired: 1 out]
        }
        frame "Find Target" {
          n81 = Equal?(x=w408, y=w409) -> (x = y?=w407:bool)
          n82 = In Range and Coerce(upper limit=25.0, x=w405, lower limit=-25.0) -> (In Range?=w402:bool)  [unwired: 1 out]
          n83 = Not(x=w402) -> (.not. x?=w401:bool)
          n84 = Unbundle By Name(w411) -> ("Time_Met"=w410:bool)
          n85 = Select(t=One_Ball_Type_Def."Turn to target", s=w410, f=w408) -> (s? t:f=w414:T2)
        }
        frame "Drive to Shoot" {
          n86 = Equal?(x=w436, y=w437) -> (x = y?=w435:bool)
          n87 = Multiply(x=w429, y=12.0) -> (x*y=w427:dbl)
          n88 = Subtract(x=w427, y="Dist_Stop_Before_Target") -> (x-y=w440:dbl)
          n89 = Greater?(x=w442, y=w440) -> (0:w443:bool)
          n90 = Select(t=One_Ball_Type_Def."Stop Three", s=w443, f=w436) -> (s? t:f=w445:T2)
          n91 = Unbundle By Name(w438) -> ("Time_Met"=w433:bool)
        }
        frame "Turn to target" {
          n92 = In Range and Coerce(upper limit=30.0, x=w465, lower limit=-30.0) -> (In Range?=w462:bool)  [unwired: 1 out]
          n93 = Equal?(x=w470, y=w469) -> (x = y?=w468:bool)
          n94 = Not(x=w462) -> (.not. x?=w459:bool)
          n95 = call "DeBounce.vi"("DB_Count"=15.0, "Value"=w459) -> ("BD_Value"=w458:bool)  [unwired: 9 in]
          n96 = Unbundle By Name(w472) -> ("Time_Met"=w456:bool)
          n97 = Select(t=One_Ball_Type_Def."Stop_After_Aim", s=w471, f=w470) -> (s? t:f=w475:T2)
        }
        frame "Shoot" {
          n98 = Equal?(x=w500, y=w499) -> (x = y?=w498:bool)
          n99 = Add(x=w490, y=5.0) -> (x+y=w496:dbl)
          n100 = Subtract(x=w490, y=5.0) -> (x-y=w493:dbl)
          n101 = In Range and Coerce(upper limit=w496, x=w491, lower limit=w493) -> (In Range?=w492:bool)  [unwired: 1 out]
          n102 = Not(x=w492) -> (.not. x?=w489:bool)
          n103 = Unbundle By Name(w502) -> ("Time_Met"=w501:bool)
          n104 = Select(t=One_Ball_Type_Def."Stop", s=w501, f=w500) -> (s? t:f=w504:T2)
        }
        frame "Stop Three" {
          n105 = Equal?(x=w527, y=w528) -> (x = y?=w523:bool)
          n106 = call "DeBounce.vi"("DB_Count"=w525, "Value"=w518) -> ("BD_Value"=w524:bool)  [unwired: 9 in]
          n107 = Unbundle By Name(w526) -> ("Time_Met"=w520:bool)
          n108 = Select(t=One_Ball_Type_Def."Shoot", s=w524, f=w527) -> (s? t:f=w531:T2)
        }
        frame "Stop_After_Aim" {
          n109 = call "DeBounce.vi"("DB_Count"=w554, "Value"=w555) -> ("BD_Value"=w553:bool)  [unwired: 9 in]
          n110 = Equal?(x=w545, y=w546) -> (x = y?=w544:bool)
          n111 = Unbundle By Name(w549) -> ("status"=w548:bool)
          n112 = Select(t=One_Ball_Type_Def."Drive to Shoot", s=w553, f=w545) -> (s? t:f=w552:T2)
        }
      }
    }
    frame Error {
      n113 = Select(t=errorcluster {"status"=FALSE, "code"=0, "source"=""}, s=w586, f=w572) -> (s? t:f=w571:errorcluster)
      n114 = Unbundle By Name(w571) -> ("status"=w570:bool, "source"=w569:string)
    }
  }
  "Rest_Gyro" <- w53
  "Rest_Encoder" <- w52
  "Drive_FWD Speed" <- w43
  "One_Ball_Auto" <- w42
  "Intake Arm Lowered" <- w41
  "Shoot" <- w37
  "Auto_Aim" <- w36
  "Drive_Enable" <- w32
  "Stage" <- w31
  "State" <- w38
  n115 = feedback-in #1(w38) -> ()
  n116 = feedback-in #2(w22) -> ()
  n117 = To Double Precision Float(number=w38) -> (double precision float=w44:dbl)
  n118 = call "Rate_Limit.vi"("Reset"=w6, "Ramp_Rate"="Ramp_Rate", "Input"=w2) -> ("Output"=→"Angle_Setpoint":dbl)  [unwired: 8 in]
  n119 = call "AutoFeed_Back.vi"("Code 4"=w14, "Error_4_En"=w18, "Code 3"=w15, "Code 2"=w16, "Error_3_En"=w19, "Error_2_En"=w20, "Code 1"=w17, "Error_1_En"=w21, "Time (ms)"=w51, "State"=w44) -> ("Feedback_State"=w13:cluster{"Time_Met":bool, "error ":errorcluster})  [unwired: 1 in]
  n120 = feedback-in #3(w13) -> ()
  n121 = Unbundle By Name(w13) -> ("error"=→"error":errorcluster)
